vi "Tempconv_Localvar.vi"() -> ()   [LabVIEW 2020]
panel:
  out "Fahrenheit":dbl(slide) scale=0.0..100.0
  out "Celsius":dbl(slide) scale=0.0..100.0
  in  "Unit":bool
  in  "Temperature":dbl
  # "When switch(unit) is on it converts celsius to fahrenheit.\nWhen switch(unit) is off it converts Fahrenheit to celsius."
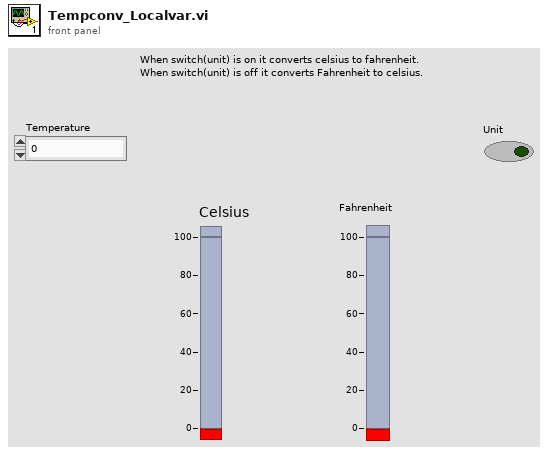
[diagram p1: front panel]
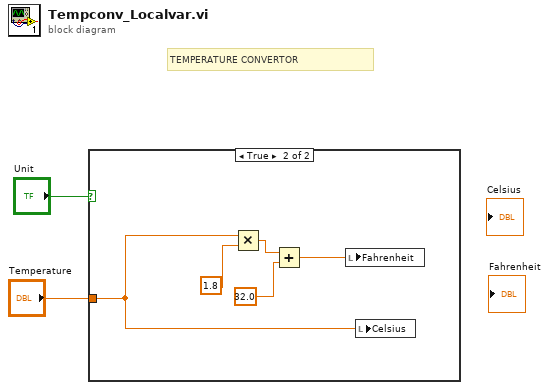
[diagram p0: block diagram]
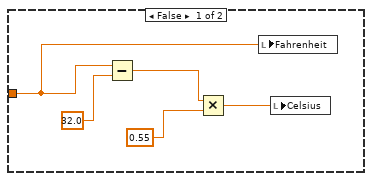
[diagram p2: hidden frame]
diagram:
  # "TEMPERATURE CONVERTOR"
  n1 = case shown="True" "Unit" {
    tunnel: "Temperature" -> [w3 w8]
    frame False {
      n2 = Subtract(x=w3, y=32.0) -> (x-y=w6:dbl)
      n3 = Multiply(x=w6, y=0.55) -> (x*y=w4:dbl)
      n4 = local write "Fahrenheit"(w3) -> ()
      n5 = local write "Celsius"(w4) -> ()
    }
    frame True {
      n6 = Multiply(x=w8, y=1.8) -> (x*y=w11:dbl)
      n7 = Add(x=w11, y=32.0) -> (x+y=w9:dbl)
      n8 = local write "Fahrenheit"(w9) -> ()
      n9 = local write "Celsius"(w8) -> ()
    }
  }
